vi "read.vi"(8 "error in (no error)":errorcluster, 10 "timeout (ms)":i32=500, 11 "DeviceInterface in":refnum<class "DeviceInterface.lvclass">) -> (0 "error out":errorcluster, 2 "Return String":string, 3 "DeviceInterface out":refnum<class "DeviceInterface.lvclass">)   [LabVIEW 2013, in "DeviceInterface.lvclass"]
doc: "Aus dem Puffer des Gerätes lesen"
uses:
  DeviceInterface.lvclass
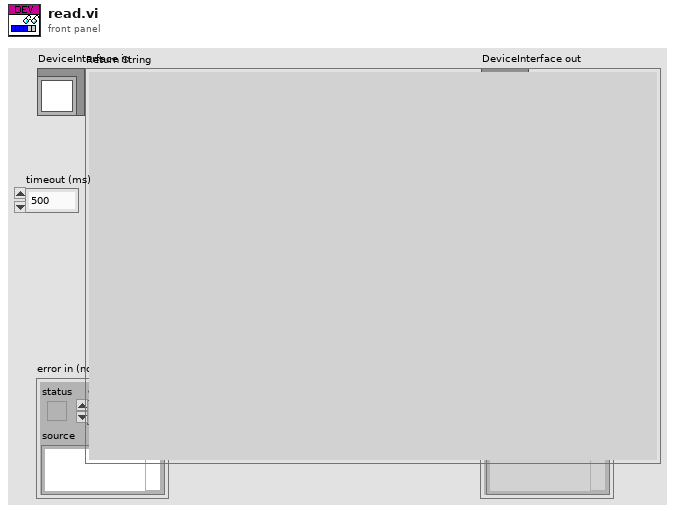
[diagram p1: front panel]
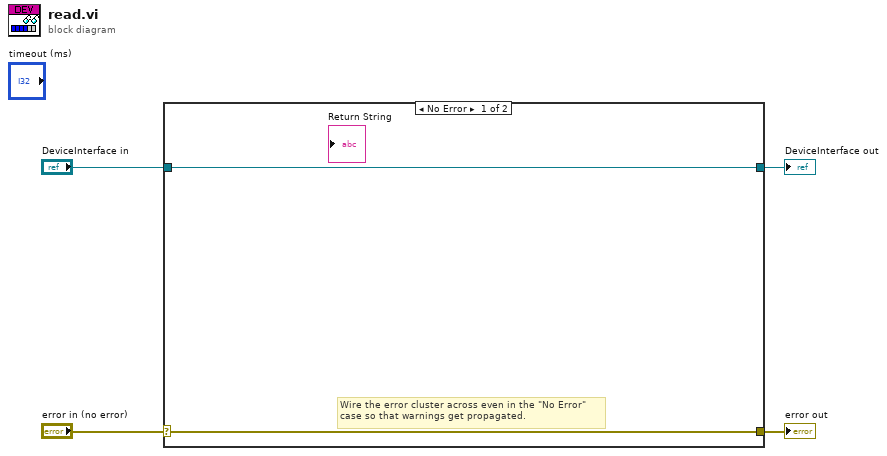
[diagram p0: block diagram]
diagram:
  n1 = case shown="No Error" "error in (no error)" {
    selector: "error in (no error)" -> [w5 w8]
    tunnel: [w5 w8] -> w3
    tunnel: [w6 w7] -> w1
    tunnel: "DeviceInterface in" -> [w6 w7]
    frame No Error {
      # "Wire the error cluster across even in the \"No Error\"\ncase so that warnings get propagated."
    }
    frame Error {
    }
  }
  "error out" <- w3
  "DeviceInterface out" <- w1
